vi "EletoMatr_1.vi"(0 "Input Array":dbl[][](array[numeric]), 5 "Input":dbl, 9 "In Row":dbl, 11 "In Column":dbl, 12 "Input Direction":bool=TRUE) -> (4 "Out Array":dbl[][](array[numeric]), 6 "Output Direction":bool=TRUE, 8 "Completed":bool=TRUE, 10 "Out Row":dbl, 15 "Out Column":dbl)   [LabVIEW 2012]
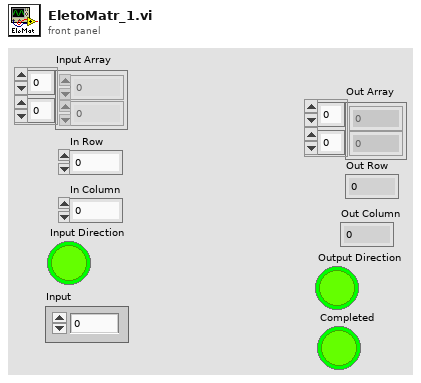
[diagram p1: front panel]
types:
  T1 = typedef "NI_Matrix.lvlib/RealMatrix.ctl" = dbl[][]
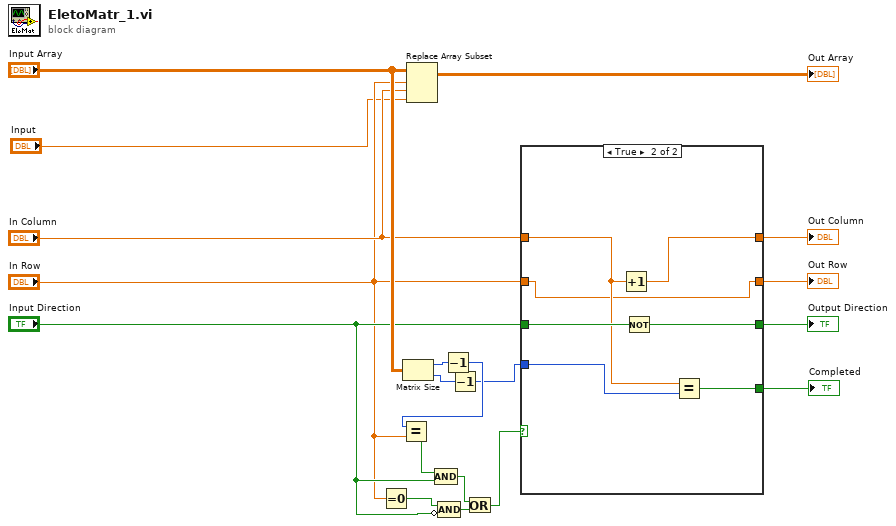
[diagram p0: block diagram]
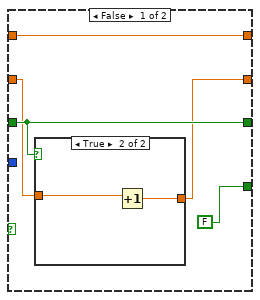
[diagram p2: hidden frame]
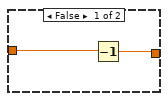
[diagram p3: hidden frame]
diagram:
  n1 = Equal To 0?(x="In Row") -> (x = 0?=w5:bool)
  n2 = Matrix Size(0:"Input Array") -> (1:w10:i32, 2:w9:i32)
  n3 = Replace Array Subset(array="Input Array", new element="Input", index (row)="In Row", index (col)="In Column") -> (→"Out Array":T1)
  n4 = Compound Arithmetic op=AND(w5, invert "Input Direction") -> (w12:bool)
  n5 = Decrement(x=w10) -> (x-1=w3:i32)
  n6 = Equal?(x=w3, y="In Row") -> (x = y?=w8:bool)
  n7 = Compound Arithmetic op=AND(w8, "Input Direction") -> (w6:bool)
  n8 = Decrement(x=w9) -> (x-1=w2:i32)
  n9 = Or(x=w6, y=w12) -> (x .or. y?=w11:bool)
  n10 = case shown="True" w11 {
    tunnel: "Input Direction" -> [w24 w35]
    tunnel: "In Row" -> [w22 w29]
    tunnel: [w20 w30] -> w18
    tunnel: "In Column" -> [w20 w31]
    tunnel: [w24 w34] -> w17
    tunnel: [w21 w29] -> w16
    tunnel: w2 -> [_ w32]
    tunnel: [FALSE w33] -> w14
    frame False {
      n11 = case shown="True" w24 {
        tunnel: [w26 w28] -> w21
        tunnel: w22 -> [w25 w27]
        frame False {
          n12 = Decrement(x=w25) -> (x-1=w26:dbl)
        }
        frame True {
          n13 = Increment(x=w27) -> (x+1=w28:dbl)
        }
      }
    }
    frame True {
      n14 = Increment(x=w31) -> (x+1=w30:dbl)
      n15 = Not(x=w35) -> (.not. x?=w34:bool)
      n16 = Equal?(x=w31, y=w32) -> (x = y?=w33:bool)
    }
  }
  "Out Row" <- w16
  "Out Column" <- w18
  "Output Direction" <- w17
  "Completed" <- w14
